vi "Set Output Voltage.vi"(8 "error in (no error)":errorcluster, 10 "Voltage [V]":dbl, 11 "Voltage Output In":refnum<class "Voltage Output.lvclass">) -> (0 "error out":errorcluster, 3 "Voltage Output Out":refnum<class "Voltage Output.lvclass">)   [LabVIEW 2020, in "High Level PSU With Tests.lvlib" / "Voltage Output.lvclass"]
uses:
  Voltage Output.lvclass
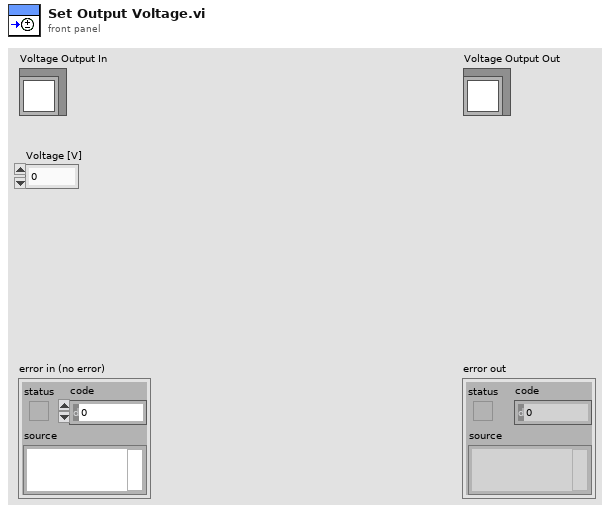
[diagram p1: front panel]
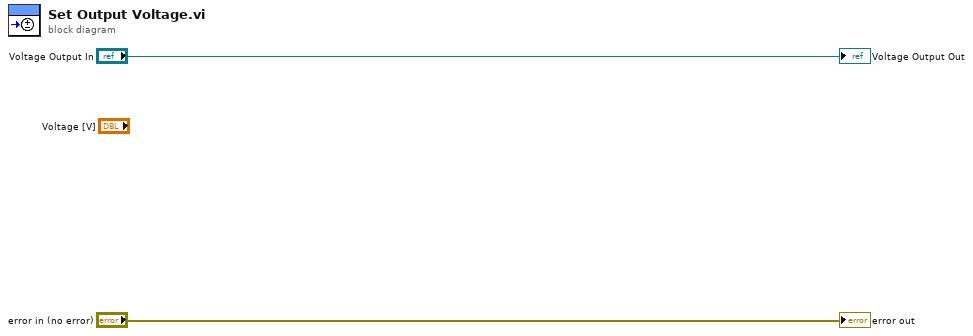
[diagram p0: block diagram]
diagram:
  "error out" <- "error in (no error)"
  "Voltage Output Out" <- "Voltage Output In"
